vi "Read Buffer.vi"(8 "error in":errorcluster, 10 "byte count":u32=100, 11 "SR 3XX HVPS in":refnum<class "SR 3XX HVPS.lvclass">) -> (0 "error out":errorcluster, 2 "ReadData":string, 3 "SR 3XX HVPS out":refnum<class "SR 3XX HVPS.lvclass">)   [LabVIEW 2014, in "SR 3XX HVPS.lvclass"]
doc: "Basic read on the HVPS located on the GPIB port designated. The read will terminate on the <B>byte count</B> specified. The default is 100 characters."
uses:
  SR 3XX HVPS.lvclass
  SR 3XX HVPS.lvclass/SR 3XX HVPS.ctl
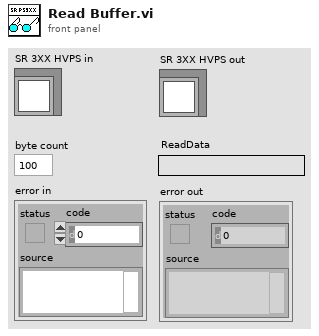
[diagram p1: front panel]
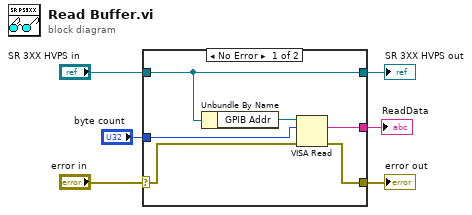
[diagram p0: block diagram]
diagram:
  n1 = case shown="No Error" "error in" {
    selector: "error in" -> [w10 w14]
    tunnel: [w9 w14] -> w5
    tunnel: [w12 w13] -> w3
    tunnel: "SR 3XX HVPS in" -> [w12 w13]
    tunnel: "byte count" -> [w8 _]
    tunnel: [w7 _] -> w1
    frame No Error {
      n2 = Unbundle By Name(w12) -> ("GPIB Addr"=w11:refnum<visa-resource-name>)
      n3 = VISA Read(VISA resource name=w11, byte count=w8, error in (no error)=w10) -> (read buffer=w7:string, error out=w9:errorcluster)  [unwired: 2 out]
    }
    frame Error {
    }
  }
  "error out" <- w5
  "SR 3XX HVPS out" <- w3
  "ReadData" <- w1
